vi "Test Get Port Status Comm.vi"(8 "error in (no error)":errorcluster, 11 "TestCase in":refnum<class "Test Get Port Status Comand.lvclass">) -> (0 "error out":errorcluster, 3 "TestCase out":refnum<class "Test Get Port Status Comand.lvclass">)   [LabVIEW 2020, in "Test Get Port Status Comand.lvclass"]
doc: "En este vi tomado como template del testExample se prueba el comando mandado para obtener el valor del puerto del microcontrolador simulado."
uses:
  Test Get Port Status Comand.lvclass
  Implementations/Simulado/Simulado.lvclass
  <vilib>/addons/_JKI Toolkits/VI Tester/TestCase.llb/TestCase.lvclass
  C:/Program Files (x86)/National Instruments/LabVIEW 2020/vi.lib/addons/_JKI Toolkits/VI Tester/TestCase.llb/TestCase.lvclass
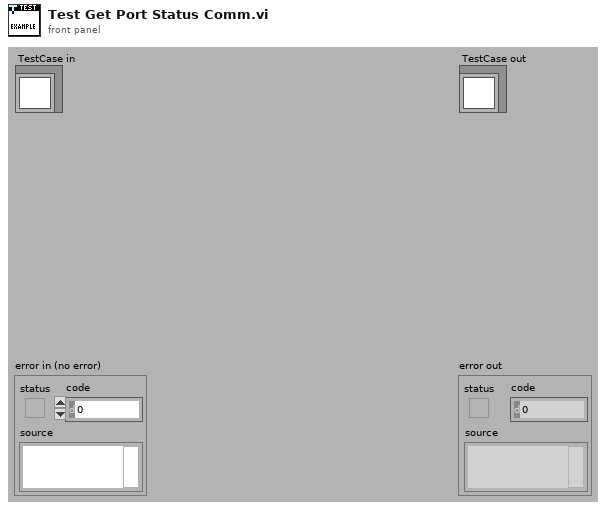
[diagram p1: front panel]
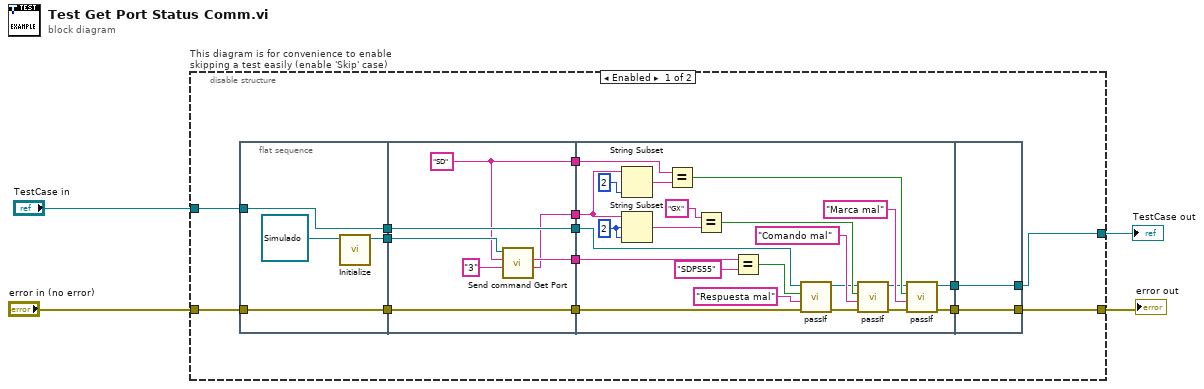
[diagram p0: block diagram]
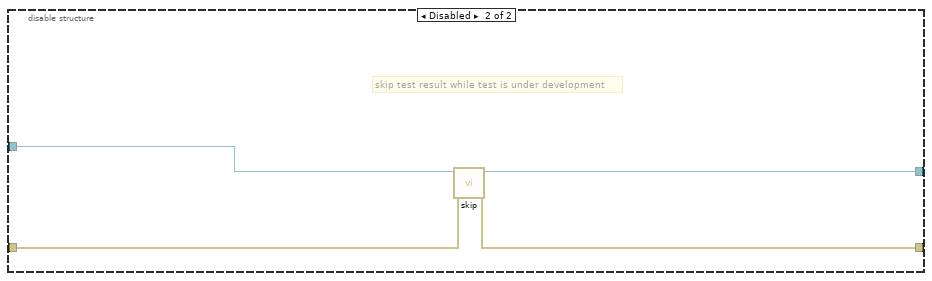
[diagram p2: hidden frame]
diagram:
  n1 = disable-structure "This diagram is for convenience to enable skipping a test easily (enable 'Skip' case)" shown="Enabled" {
    disable-tunnel: "TestCase in" -> [w9 w58]
    disable-tunnel: [w7 w56] -> w1
    disable-tunnel: [w6 w57] -> w3
    disable-tunnel: "error in (no error)" -> [w8 w55]
    frame Enabled {
      n2 = flat-sequence {
        tunnel: w9 -> [w22]
        tunnel: [w22] -> w18
        tunnel: w8 -> [w21]
        tunnel: [w21] -> w17
        tunnel: [w19] -> w16
        tunnel: [w29] -> w15
        tunnel: w18 -> [w29]
        tunnel: [w28] -> w14
        tunnel: w17 -> [w28]
        tunnel: w16 -> [w27]
        tunnel: [w24] -> w13
        tunnel: [w26] -> w12
        tunnel: [w23] -> w5
        tunnel: [w49] -> w11
        tunnel: w15 -> [w36]
        tunnel: [w48] -> w10
        tunnel: w14 -> [w34]
        tunnel: w13 -> [w38]
        tunnel: w12 -> [w50]
        tunnel: w5 -> [w30]
        tunnel: [w54] -> w7
        tunnel: w11 -> [w54]
        tunnel: [w53] -> w6
        tunnel: w10 -> [w53]
        frame #0 {
          n3 = call-dynamic "Initialize.vi"("object in"=refnum<class "Simulado.lvclass"> refnum ("Simulado.lvclass")) -> ("object out"=w19:refnum<class "Simulado.lvclass">)  [unwired: 9 in, 1 out]
        }
        frame #1 {
          w26 = "SD" ("Marca")
          n4 = call-dynamic "Send command Get Port.vi"("Puerto"="3", "Marca"=w26, "Simulado in"=w27) -> ("Command"=w23:string, "Expected response"=w24:string)  [unwired: 5 in, 2 out]
        }
        frame #2 {
          w45 = 2 ("length (rest)")
          n5 = String Subset(string=w30, length (rest)=2 ("length (rest)")) -> (substring=w51:string)  [unwired: 1 in]
          n6 = String Subset(string=w30, offset (0)=w45, length (rest)=w45) -> (substring=w44:string)
          n7 = Equal?(x=w50, y=w51) -> (x = y?=w47:bool)
          n8 = Equal?(x="GX", y=w44) -> (x = y?=w40:bool)
          n9 = Equal?(x=w38, y="SDPS55") -> (x = y?=w32:bool)
          n10 = call-dynamic "passIf.vi"("error in (no error)"=w34, "message (\"\")"="Respuesta mal" ("message (\"\")"), "pass"=w32, "TestCase in"=w36) -> ("error out"=w33:errorcluster, "TestCase out"=w35:refnum<class "Test Get Port Status Comand.lvclass">)  [unwired: 6 in]
          n11 = call-dynamic "passIf.vi"("error in (no error)"=w33, "message (\"\")"="Comando mal" ("message (\"\")"), "pass"=w40, "TestCase in"=w35) -> ("error out"=w41:errorcluster, "TestCase out"=w42:refnum<class "Test Get Port Status Comand.lvclass">)  [unwired: 6 in]
          n12 = call-dynamic "passIf.vi"("error in (no error)"=w41, "message (\"\")"="Marca mal" ("message (\"\")"), "pass"=w47, "TestCase in"=w42) -> ("error out"=w48:errorcluster, "TestCase out"=w49:refnum<class "Test Get Port Status Comand.lvclass">)  [unwired: 6 in]
        }
        frame #3 {
        }
      }
    }
    frame Disabled {
      # "skip test result while test is under development"
      n13 = call <vilib>:"skip.vi"("error in (no error)"=w55, "TestCase in"=w58) -> ("error out"=w57:errorcluster, "TestCase out"=w56:refnum<class "Test Get Port Status Comand.lvclass">)  [unwired: 8 in]
    }
  }
  "error out" <- w3
  "TestCase out" <- w1
